vi "Download.vi"(6 "Value":variant, 8 "error in":errorcluster, 9 "Multiplexer":cluster{"Index":u16, "Sub-Index":u8} {"Index" format="%.0x"}, 10 "Node-ID":u8, 11 "CANopen Master in":refnum<class "CANopen Master.lvclass">) -> (0 "error out":errorcluster, 2 "Success?":bool, 3 "CANopen Master out":refnum<class "CANopen Master.lvclass">)   [LabVIEW 2024, in "CANopen Master.lvlib" / "CANopen Master.lvclass"]
uses:
  CANopen Master.lvclass
  CANopen Master.lvclass/CANopen Master.ctl
  SDO Manager/SDO Manager.lvclass
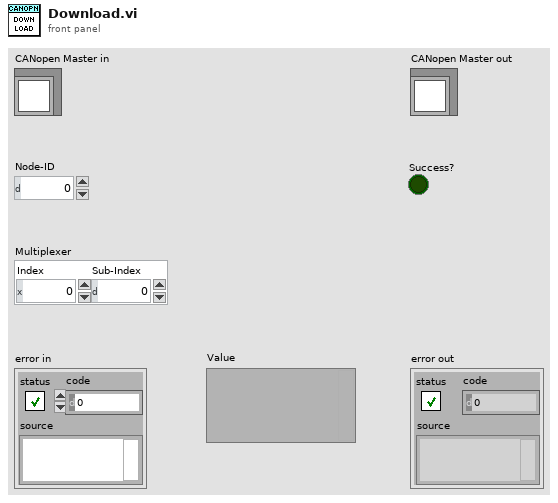
[diagram p1: front panel]
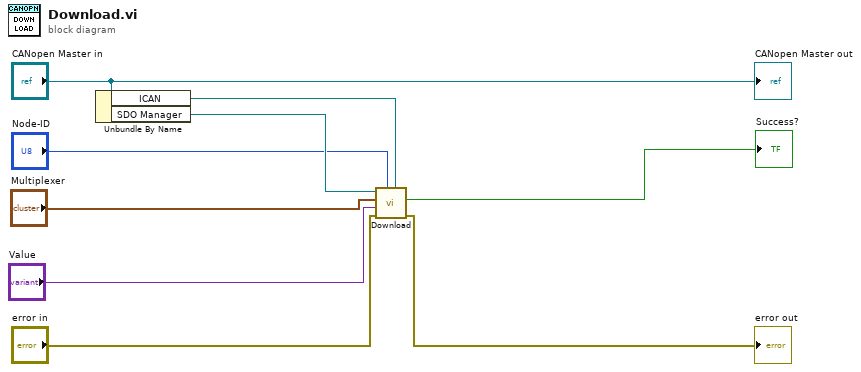
[diagram p0: block diagram]
diagram:
  n1 = Unbundle By Name("CANopen Master in") -> ("ICAN"=w7:refnum<class "ICAN.lvclass">, "SDO Manager"=w8:refnum<class "SDO Manager.lvclass">)
  n2 = call "Download.vi"("ICAN"=w7, "Node-ID"="Node-ID", "error in"="error in", "Value"="Value", "Multiplexer"="Multiplexer", "SDO Manager in"=w8) -> ("error out"=→"error out":errorcluster, "Success?"=→"Success?":bool)  [unwired: 3 in, 1 out]
  "CANopen Master out" <- "CANopen Master in"
